vi "Build Battery Switch Section from XML.vi"(6 "Channels":refnum<k24>[](array[refnum]), 8 "error in (no error)":errorcluster, 9 "Card Position in":T1 {"Slot #" max=15}, 10 "Name in":string, 11 "Node Ptr in":u64) -> (0 "error out":errorcluster)   [LabVIEW 2014, in "SLSC configuration System Explorer.lvlib"]
uses:
  SLSC configuration System Explorer.lvlib
  Type Defs/Card Position.ctl
  Shared/SPI Utility/Slot #.ctl
  C:/Files/Custom VeriStand Development/DET-SPI-Tool/XML Deserializer/SLSC Deserializer/SLSC Deserializer/bin/Release/SLSC Deserializer.dll
  XML Deserializer/SLSC Deserializer/SLSC Deserializer/bin/Release/SLSC Deserializer.dll
  <vilib>/NI Veristand/Custom Device API/Custom Device Channel.ctl
  <vilib>/NI Veristand/Custom Device API/Custom Device Channel Type.ctl
  Shared/Constants.vi
  <vilib>/NI Veristand/Custom Device API/Set Item Property (U16).vi
  <vilib>/NI Veristand/Custom Device API/Custom Device API.lvlib
  Shared/SLSC configuration Shared.lvlib
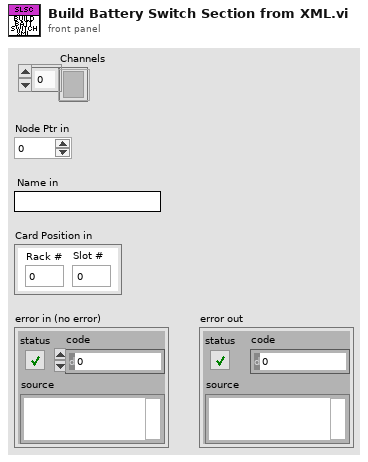
[diagram p1: front panel]
types:
  T1 = typedef "SLSC configuration Shared.lvlib/Card Position.ctl" = cluster{"Rack #":u8, "Slot #":T2}
  T2 = typedef "SLSC configuration Shared.lvlib/Slot #.ctl" = u8
  T3 = typedef "Custom Device API.lvlib/Custom Device Channel Type.ctl" = enum16{"Input", "Output"}
  T4 = typedef "Custom Device API.lvlib/Custom Device Channel.ctl" = cluster{"Type":T3, "Units":string, "Default Value":dbl, "Faultable":bool, "Scalable":bool}
  T5 = typedef "Custom Device API.lvlib/Custom Device Item Ref.ctl" = u64
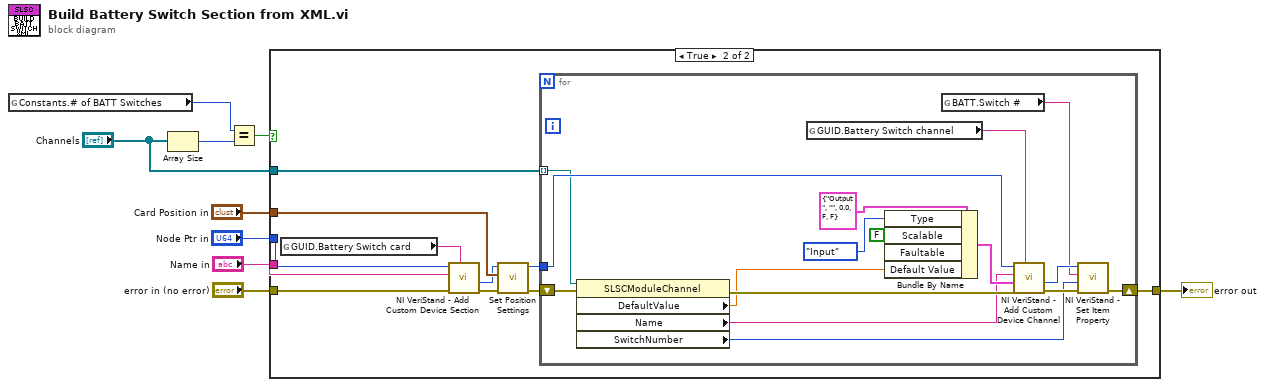
[diagram p0: block diagram]
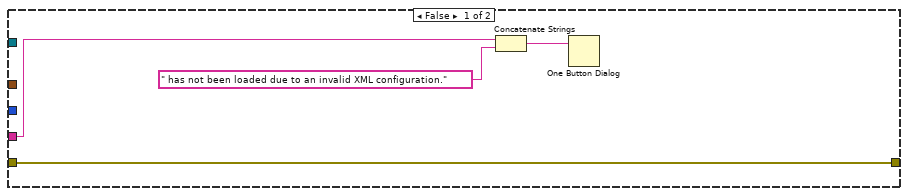
[diagram p2: hidden frame]
diagram:
  n1 = global read "Constants.vi" "Constants.# of BATT Switches"() -> (w3:u8)
  n2 = Array Size(array="Channels") -> (size(s)=w4:i32)
  n3 = Equal?(x=w3, y=w4) -> (x = y?=w1:bool)
  n4 = case shown="True" w1 {
    tunnel: "Name in" -> [w13 w24]
    tunnel: "Card Position in" -> [_ w23]
    tunnel: "Node Ptr in" -> [_ w22]
    tunnel: "error in (no error)" -> [w10 w21]
    tunnel: [w10 w15] -> w5
    tunnel: "Channels" -> [_ w14]
    frame False {
      n5 = Concatenate Strings(w13, " has not been loaded due to an invalid XML configuration." ("string")) -> (w11:string)
      n6 = One Button Dialog(message=w11) -> ()  [unwired: 1 in, 1 out]
    }
    frame True {
      n7 = global read "Constants.vi" "GUID.Battery Switch card"() -> (w20:string)
      n8 = call <vilib>:"NI VeriStand - Add Custom Device Section.vi"("GUID (Default Section)"=w20, "error in (no error)"=w21, "Section Name"=w24, "Parent Ref in"=w22) -> ("error out"=w19:errorcluster, "Section Ptr"=w18:T5)  [unwired: 4 in, 2 out]
      n9 = call "Set Position Settings.vi"("error in (no error)"=w19, "Card Position"=w23, "Item Ref in"=w18) -> ("error out"=w17:errorcluster, "Item Ref out"=w16:T5)  [unwired: 7 in]
      n10 = for {
        shift-right: [w31] -> w15
        shift-left: w17 -> [w30]
        tunnel: w16 -> [w34]
        tunnel: w14 -> [w29] mode=indexing
        w37 = FALSE ("Scalable")
        n11 = property class="SLSCModuleChannel"(reference=w29, error in=w30) -> (error out=w28:errorcluster, "DefaultValue"=w25:dbl, "Name"=w26:string, "SwitchNumber"=w27:u8)  [unwired: 1 out]
        n12 = global read "Constants.vi" "GUID.Battery Switch channel"() -> (w36:string)
        n13 = Bundle By Name(cluster=T4 {"Type"=enum."Output", "Units"="", "Default Value"=0.0, "Faultable"=FALSE, "Scalable"=FALSE} ("Channel"), "Type"=Custom_Device_Channel_Type."Input", "Scalable"=w37, "Faultable"=w37, "Default Value"=w25) -> (w39:T4)
        n14 = global read "Constants.vi" "BATT.Switch #"() -> (w32:string)
        n15 = call <vilib>:"NI VeriStand - Add Custom Device Channel.vi"("GUID (Default Channel)"=w36, "error in (no error)"=w28, "Channel"=w39, "Channel Name"=w26, "Parent Ref in"=w34) -> ("error out"=w35:errorcluster, "Channel Ref"=w33:T5)  [unwired: 3 in, 2 out]
        n16 = call-poly <vilib>:"NI VeriStand - Set Item Property.vi"("error in (no error)"=w35, "Value"=w27, "Property Name"=w32, "Item Ref in"=w33) -> ("error out"=w31:errorcluster)  [unwired: 5 in, 2 out]
      }
    }
  }
  "error out" <- w5
